vi "Command_to_webserver.vi"(8 "Error In":errorcluster, 9 "JSON post command":string, 10 "URL Command to Logout":string, 11 "https client handle in ref":T1) -> (0 "Error Out":errorcluster, 1 "Header of response for debug purpose":string, 2 "Body of response":string, 3 "https client handle out ref":T1, 4 "Reponse time":u32)   [LabVIEW 2017]
doc: "Send POST command to webserver:\n1. This Sub VI accepts command and string input \n2. Both the values will be sent to webserver for processing\n3. It captures the response from the webserver and pass to next module for test result processing"
uses:
  <vilib>/httpClient/ClientHandle.ctl
  <vilib>/httpClient/POSTBuffer.vi
  <vilib>/httpClient/LabVIEWHTTPClient.lvlib
panel:
  # "RESPONSE FROM WEBSERVER"
  # "LOGOUT"
  # "ERROR"
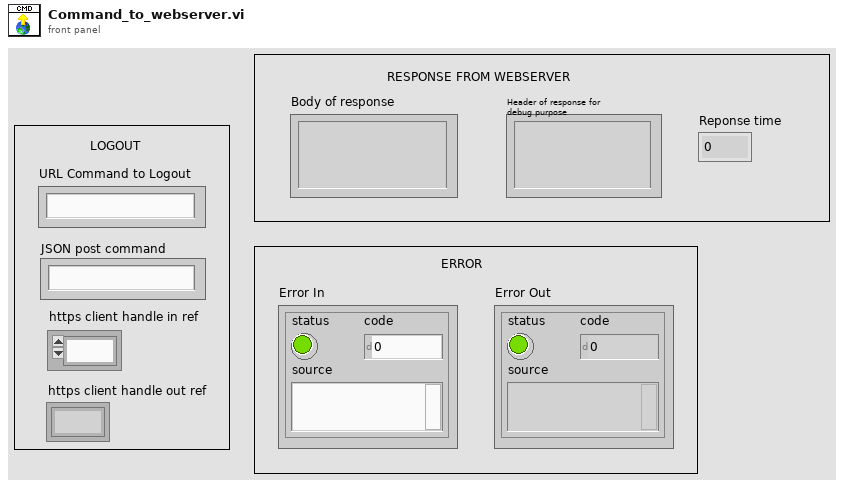
[diagram p1: front panel]
types:
  T1 = typedef "LabVIEWHTTPClient.lvlib/ClientHandle.ctl" = refnum<k1>
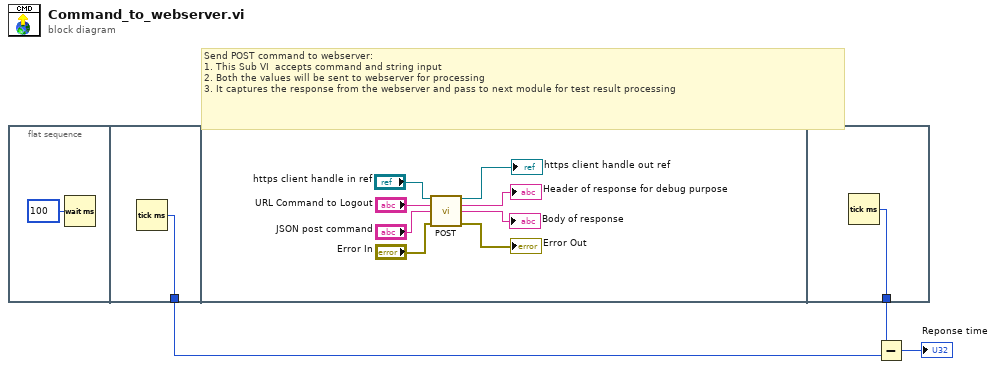
[diagram p0: block diagram]
diagram:
  # "Send POST command to webserver:\n1. This Sub VI  accepts command and string input \n2. Both the values will be sent to webserver for processing\n3. It captures the response from the webserver and pass to next module for test result processing"
  n1 = flat-sequence {
    tunnel: [w5] -> w3
    tunnel: [w14] -> w2
    frame #0 {
      n2 = Wait (ms)(milliseconds to wait=u32 100) -> ()  [unwired: 1 out]
    }
    frame #1 {
      n3 = Tick Count (ms)() -> (millisecond timer value=w5:u32)
    }
    frame #2 {
      n4 = call-poly <vilib>:"POST.vi"("client handle"="https client handle in ref", "url"="URL Command to Logout", "buffer"="JSON post command", "error in (no error)"="Error In") -> ("client handle out"=→"https client handle out ref":T1, "headers"=→"Header of response for debug purpose":string, "body"=→"Body of response":string, "error out"=→"Error Out":errorcluster)  [unwired: 8 in]
    }
    frame #3 {
      n5 = Tick Count (ms)() -> (millisecond timer value=w14:u32)
    }
  }
  n6 = Subtract(x=w2, y=w3) -> (x-y=→"Reponse time":u32)
